vi "setXAxisConversionType.vi"(8 "error in (no error)":errorcluster, 10 "Enum":T1, 11 "CCD in":refnum<class "CCD.lvclass">) -> (0 "error out":errorcluster, 1 "ID":i32, 2 "results-JSON string":string, 3 "CCD out":refnum<class "CCD.lvclass">)   [LabVIEW 2023, in "CCD.lvclass"]
uses:
  CCD.lvclass
  CCD.lvclass/CCD.ctl
  20f7d3bd-08ac-4524-9bed-df36c1da25a0.vi
  GenericDevice/GenericDevice.lvclass
  3e78960f-3857-40ea-b6b5-da67a5e4625c.vi
  <vilib>/IlluminatedG/lv-web-crypto/lv-json/JSON/JSON.lvlib
  XAxisConversionTypeEnum.ctl
panel:
  # "Connector Pane"
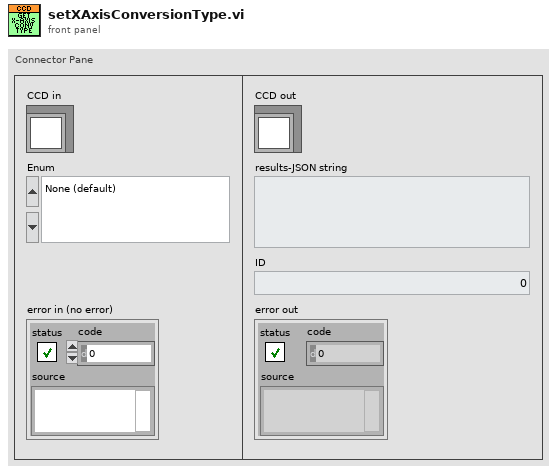
[diagram p1: front panel]
types:
  T1 = typedef "CCD.lvclass/XAxisConversionTypeEnum.ctl" = enum16{"None (default)", "CCD FIT parameters contained in the CCD firmware", "Mono Wavelength parameters contained in the icl_settings.ini file"}
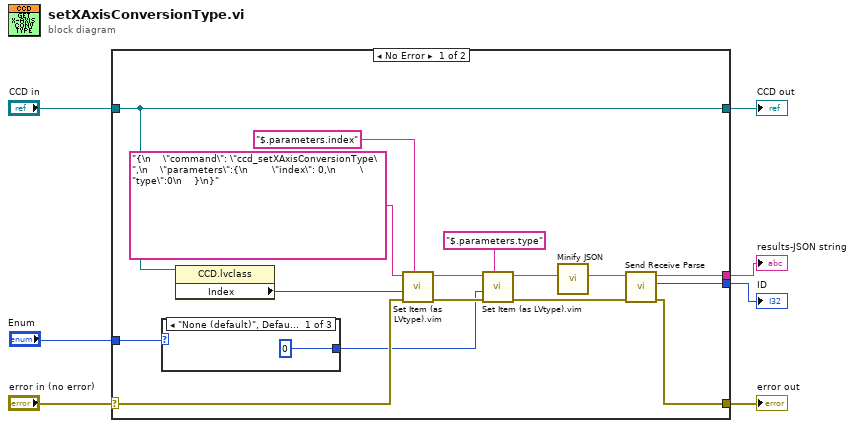
[diagram p0: block diagram]
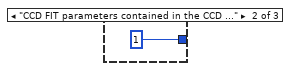
[diagram p2: hidden frame]
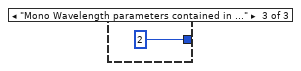
[diagram p3: hidden frame]
diagram:
  n1 = case shown="No Error" "error in (no error)" {
    selector: "error in (no error)" -> [w19 w28]
    tunnel: [w14 w28] -> w6
    tunnel: [w21 w27] -> w4
    tunnel: "CCD in" -> [w21 w27]
    tunnel: "Enum" -> [w9 _]
    tunnel: [w13 _] -> w2
    tunnel: [w12 _] -> w1
    frame No Error {
      n2 = case shown="\"None (default)\", Default" w9 {
        tunnel: [0 1 2] -> w8
        frame "None (default)", Default {
        }
        frame "CCD FIT parameters contained in the CCD firmware" {
        }
        frame "Mono Wavelength parameters contained in the icl_settings.ini file" {
        }
      }
      n3 = property class="CCD.lvclass"(reference=w21) -> ("Index"=w20:i32)  [unwired: 1 in, 2 out]
      n4 = call "Set Item (as LVtype).vim"("$Path or Item Name"="$.parameters.index", "error in (no error)"=w19, "Anything"=w20, "JSON"="{\n    \"command\": \"ccd_setXAxisConversionType\",\n    \"parameters\":{\n        \"index\": 0,\n        \"type\":0\n    }\n}") -> ("error out"=w17:errorcluster, "<JSON>"=w18:string)  [unwired: 4 in, 1 out]
      n5 = call "Set Item (as LVtype).vim"("$Path or Item Name"="$.parameters.type", "error in (no error)"=w17, "Anything"=w8, "JSON"=w18) -> ("error out"=w16:errorcluster, "<JSON>"=w11:string)  [unwired: 4 in, 1 out]
      n6 = call <vilib>:"Minify JSON.vi"("JSON String"=w11) -> ("Minified JSON"=w10:string)  [unwired: 10 in]
      n7 = call "Send Receive Parse.vi"("error in"=w16, "<JSON>"=w10) -> ("error out"=w14:errorcluster, "ID"=w12:i32, "results-JSON string"=w13:string)  [unwired: 7 in]
    }
    frame Error {
    }
  }
  "error out" <- w6
  "CCD out" <- w4
  "results-JSON string" <- w2
  "ID" <- w1
